vi "斯坦道XML解析.vi"(9 "工作状态":u16, 10 "添加的路径":path, 11 "参数簇":cluster{"id":u16, "flowid":dbl, "range":dbl}={"id"=1, "flowid"=0.0, "range"=0.0}) -> (1 "简易步骤名称":string, 2 "步骤时间":string[](array[string]), 3 "步骤名":string[](array[string]))   [LabVIEW 2016, in "斯坦道氟化物.lvlib"]
uses:
  <vilib>/xml/Load XML File.vi
  <vilib>/xml/Close Reference(Node).vi
  C:/Program Files (x86)/National Instruments/LabVIEW 2016/resource/objmgr/DOMUserDefRef.rc
  <vilib>/xml/NI_XML.lvlib
panel:
  out "连接的字符串":string
  out "大小":i32
  out "XML字符串":string="<?xml version=\"1.0\" encoding=\"ISO-8859-1\"?>\n<bookstore>\n<book ISBN=\"978-0545128285\">\n  <title lang=\"en\">The Tales of Beedle the Bard</title>\n  <author>J. K. Rowling</author>\n  <year>2008</year>\n  <price>12.99</price>\n</book>\n<book ISBN=\"978-0316160209\">\n  <title lang=\"en\">Eclipse</title>\n  <author>Stephenie Meyer</author>\n  <year>2007</year>\n  <price>19.99</price>\n</book>\n<book ISBN=\"978-0316067928\">\n  <title lang=\"en\">Breaking Dawn</title>\n  <author>Stephenie Meyer</author>\n  <year>2008</year>\n  <price>22.99</price>\n</book>\n<book ISBN=\"978-0316017923\">\n  <title lang=\"en\">Outliers: The Story of Success</title>\n  <author>Malcolm Gladwell</author>\n  <year>2008</year>\n  <price>27.99</price>\n</book>\n<book ISBN=\"978-0596007645\">\n  <title lang=\"en\">XML in a Nutshell</title>\n  <author>Elliotte Rusty Harold</author>\n  <author>W. Scott Means</author>\n  <year>2004</year>\n  <price>39.95</price>\n</book>\n</bookstore>"
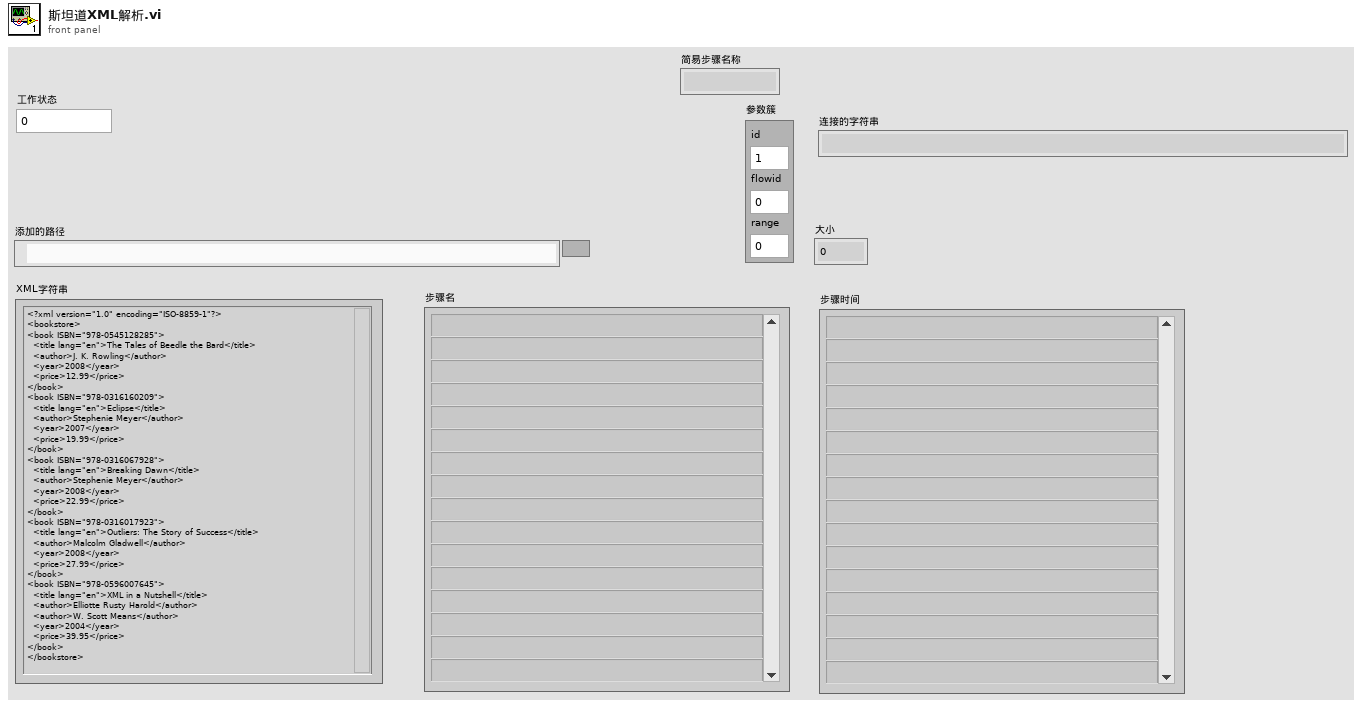
[diagram p1: front panel]
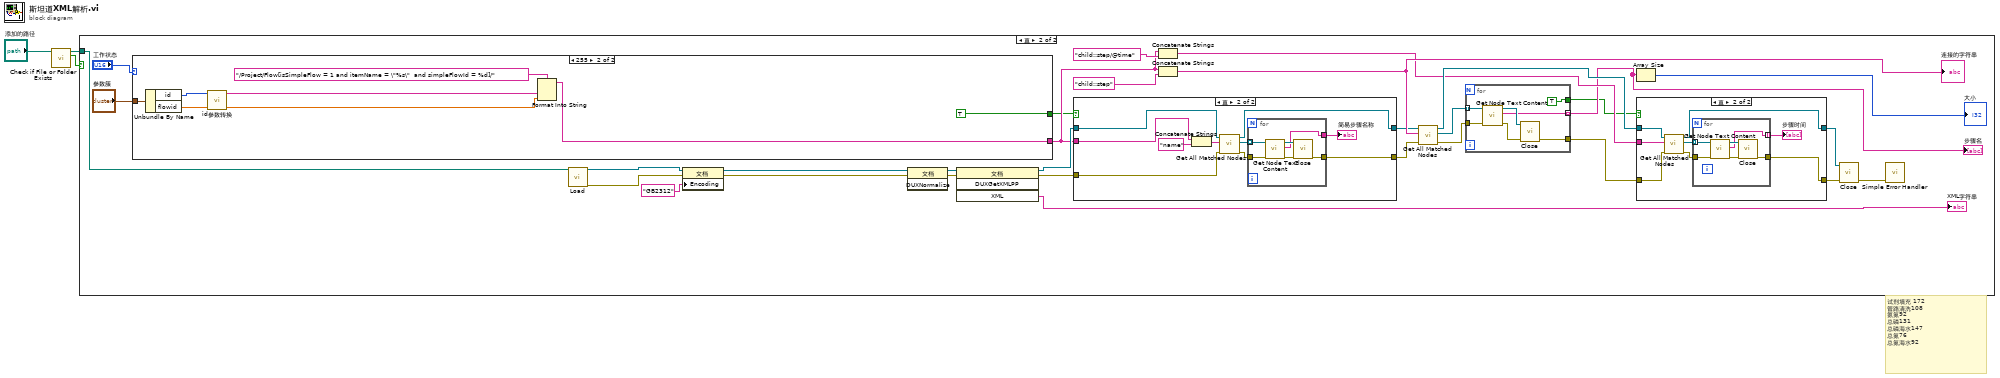
[diagram p0: block diagram]
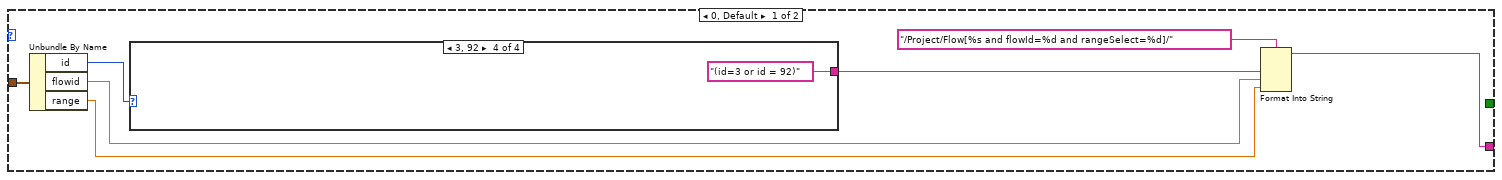
[diagram p5: hidden frame]
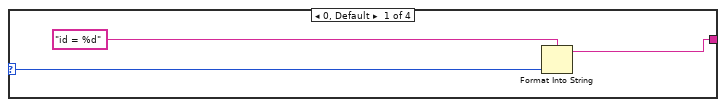
[diagram p6: hidden frame]
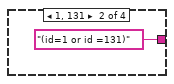
[diagram p7: hidden frame]
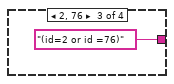
[diagram p8: hidden frame]
diagram:
  # "试剂填充 172 \n管路清洗108\n氨氮92\n总磷131\n总磷海水147\n总氮76\n总氮海水92"
  n1 = call <vilib>:"Check if File or Folder Exists.vi"("path"="添加的路径") -> ("file or folder exists?"=w1:bool, "dup path"=w2:path)  [unwired: 8 in, 1 out]
  n2 = case shown="真" w1 {
    tunnel: w2 -> [_ w22]
    frame False {
    }
    frame True {
      n3 = case shown="255" "工作状态" {
        tunnel: "参数簇" -> [w75 w88]
        tunnel: [w71 w85] -> w7
        tunnel: [_ TRUE] -> w5
        frame 0, Default {
          n4 = Unbundle By Name(w75) -> ("id"=w70:u16, "flowid"=w73:dbl, "range"=w72:dbl)
          n5 = case shown="3, 92" w70 {
            selector: w70 -> [w77 _ _ _]
            tunnel: [w76 "(id=1 or id =131)" ("输入 4") "(id=2 or id =76)" ("输入 4") "(id=3 or id = 92)" ("输入 4")] -> w69
            frame 0, Default {
              n6 = Format Into String(format string="id = %d" ("格式字符串"), w77) -> (resulting string=w76:string)  [unwired: 2 in, 1 out]
            }
            frame 1, 131 {
            }
            frame 2, 76 {
            }
            frame 3, 92 {
            }
          }
          n7 = Format Into String(format string="/Project/Flow[%s and flowId=%d and rangeSelect=%d]/" ("XPath expression"), w69, w73, w72) -> (resulting string=w71:string)  [unwired: 2 in, 1 out]
        }
        frame 255 {
          n8 = Unbundle By Name(w88) -> ("id"=w84:u16, "flowid"=w86:dbl)
          n9 = call "id参数转换.vi"("id"=w84) -> ("table输出"=w83:string)  [unwired: 9 in, 1 out]
          n10 = Format Into String(format string="/Project/Flow[isSimpleFlow = 1 and itemName = \"%s\"  and simpleFlowId = %d]/" ("XPath expression"), w83, w86) -> (resulting string=w85:string)  [unwired: 2 in, 1 out]
        }
      }
      n11 = call-poly <vilib>:"Load.vi"("path to XML document"=w22) -> ("DOM document out"=w30:refnum<k20>, "error out"=w29:errorcluster)  [unwired: 12 in, 1 out]
      n12 = property on="属性节点" class="文档"(reference=w30, error in=w29, "Encoding"="GB2312" ("文档编码")) -> (reference out=w28:refnum<k20>, error out=w27:errorcluster)
      n13 = invoke on="Invoke Node" class="文档" method="DUXNormalize"(reference=w28, error in=w27) -> (reference out=w25:refnum<k20>, error out=w26:errorcluster)  [unwired: 1 in, 1 out]
      n14 = invoke on="Invoke Node" class="文档" method="DUXGetXMLPP"(reference=w25, error in=w26) -> (reference out=w10:refnum<k20>, error out=w9:errorcluster, "XML"=→"XML字符串":string)  [unwired: 2 in, 1 out]
      n15 = case shown="真" w5 {
        tunnel: w10 -> [w52 w62]
        tunnel: w9 -> [w51 w61]
        tunnel: [w52 w60] -> w8
        tunnel: w7 -> [_ w58]
        tunnel: [w51 w54] -> w6
        frame False {
        }
        frame True {
          n16 = Concatenate Strings(w58, "name" ("输入 4")) -> (w57:string)
          n17 = call <vilib>:"Get All Matched Nodes.vi"("error in (no error)"=w61, "XPath expression"=w57, "node in"=w62) -> ("error out"=w55:errorcluster, "node result array"=w56:refnum<k20>[], "node out"=w60:refnum<k20>)  [unwired: 6 in]
          n18 = for {
            tunnel: w55 -> [w68]
            tunnel: [w65] -> w53
            tunnel: w56 -> [w64] mode=indexing
            tunnel: [w63] -> w54
            n19 = call <vilib>:"Get Node Text Content.vi"("error in (no error)"=w68, "node in"=w64) -> ("error out"=w66:errorcluster, "node text"=w65:string, "node out"=w67:refnum<k20>)  [unwired: 7 in]
            n20 = call-poly <vilib>:"Close.vi"("error in (no error)"=w66, "node"=w67) -> ("error out"=w63:errorcluster)  [unwired: 7 out]
          }
          "简易步骤名称" <- w53
        }
      }
      n21 = Concatenate Strings(w7, "child::step/@time" ("输入 4")) -> (w14:string)
      n22 = Concatenate Strings(w7, "child::step" ("输入 4")) -> (w16:string)
      "连接的字符串" <- w16
      n23 = call <vilib>:"Get All Matched Nodes.vi"("error in (no error)"=w6, "XPath expression"=w16, "node in"=w8) -> ("error out"=w21:errorcluster, "node result array"=w20:refnum<k20>[], "node out"=w19:refnum<k20>)  [unwired: 6 in]
      n24 = for {
        tunnel: w21 -> [w95]
        tunnel: [w92] -> w13 mode=indexing
        tunnel: w20 -> [w91] mode=indexing
        tunnel: [w90] -> w18
        tunnel: [TRUE] -> w4
        n25 = call <vilib>:"Get Node Text Content.vi"("error in (no error)"=w95, "node in"=w91) -> ("error out"=w93:errorcluster, "node text"=w92:string, "node out"=w94:refnum<k20>)  [unwired: 7 in]
        n26 = call-poly <vilib>:"Close.vi"("error in (no error)"=w93, "node"=w94) -> ("error out"=w90:errorcluster)  [unwired: 7 out]
      }
      "步骤名" <- w13
      n27 = Array Size(array=w13) -> (size(s)=→"大小":i32)
      n28 = case shown="真" w4 {
        tunnel: [w35 w44] -> w24
        tunnel: [w36 w43] -> w23
        tunnel: w19 -> [w36 w40]
        tunnel: w18 -> [w35 w39]
        tunnel: w14 -> [_ w37]
        frame False {
        }
        frame True {
          n29 = call <vilib>:"Get All Matched Nodes.vi"("error in (no error)"=w39, "XPath expression"=w37, "node in"=w40) -> ("error out"=w42:errorcluster, "node result array"=w41:refnum<k20>[], "node out"=w43:refnum<k20>)  [unwired: 6 in]
          n30 = for {
            tunnel: w42 -> [w50]
            tunnel: [w47] -> w38 mode=indexing
            tunnel: w41 -> [w46] mode=indexing
            tunnel: [w45] -> w44
            n31 = call <vilib>:"Get Node Text Content.vi"("error in (no error)"=w50, "node in"=w46) -> ("error out"=w48:errorcluster, "node text"=w47:string, "node out"=w49:refnum<k20>)  [unwired: 7 in]
            n32 = call-poly <vilib>:"Close.vi"("error in (no error)"=w48, "node"=w49) -> ("error out"=w45:errorcluster)  [unwired: 7 out]
          }
          "步骤时间" <- w38
        }
      }
      n33 = call-poly <vilib>:"Close.vi"("error in (no error)"=w24, "node"=w23) -> ("error out"=w34:errorcluster)  [unwired: 7 out]
      n34 = call <vilib>:"Simple Error Handler.vi"("error in (no error)"=w34) -> ()  [unwired: 4 in, 5 out]
    }
  }
